vi "init.vi"(8 "error in (no error)":errorcluster, 10 "Torque Value":refnum<data-value>, 11 "Torque Transducer in":refnum<class "Torque Transducer.lvclass">) -> (0 "error out":errorcluster, 3 "Torque Transducer out":refnum<class "Torque Transducer.lvclass">)   [LabVIEW 2025, in "Torque Transducer.lvclass"]
uses:
  Torque Transducer.lvclass
  Torque Transducer.lvclass/Torque Transducer.ctl
  <vilib>/DAQmx/create/channels.llb/DAQmx Create Channel (AI-Torque-Bridge-Two-Point-Linear).vi
  <vilib>/DAQmx/configure/timing.llb/DAQmx Timing (Sample Clock).vi
panel:
  in  "units":i32(ring)=15882 items=["Nm"=15881, "oz-in"=15882, "lb-in"=15883, "lb-ft"=15884, "From Custom Scale"=10065]
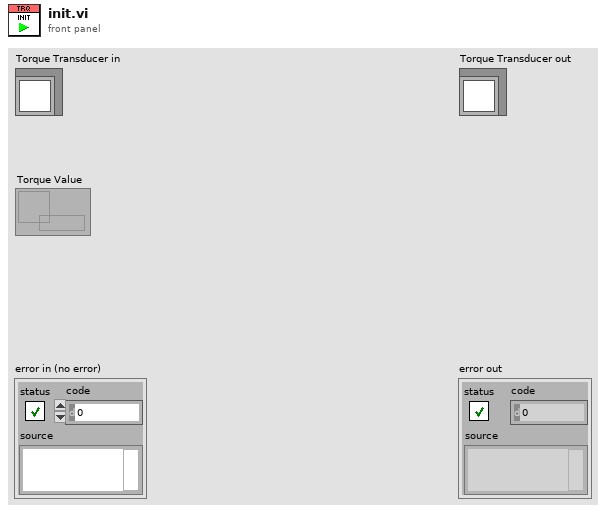
[diagram p1: front panel]
types:
  T1 = cluster{"first electrical value":dbl, "second electrical value":dbl, "electrical units":i32, "first physical value":dbl, "second physical value":dbl, "physical units":i32}
  T2 = cluster{"bridge configuration":i32, "voltage excitation source":i32, "voltage excitation value":dbl, "nominal bridge resistance":dbl}
  T3 = typedef "LVStringsAndValuesArrayTypeDef_I32.ctl" = cluster{"String":string, "Value":i32}[]
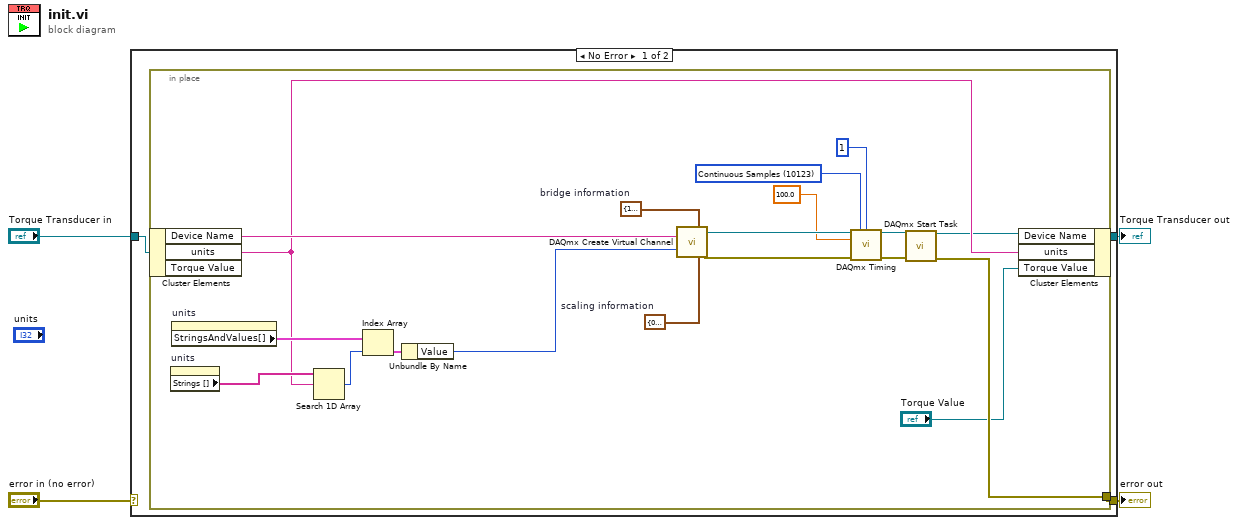
[diagram p0: block diagram]
diagram:
  n1 = case shown="No Error" "error in (no error)" {
    selector: "error in (no error)" -> [_ w28]
    tunnel: [w5 w28] -> w3
    tunnel: [w6 w27] -> w1
    tunnel: "Torque Transducer in" -> [w7 w27]
    frame No Error {
      n2 = in-place {
        in-place-border: [w9] -> w5
        w12 = 10123 items=["Finite Samples"=10178, "Continuous Samples"=10123, "Hardware Timed Single Point"=12522] ("sample mode")
        w19 = T1 {"first electrical value"=0.0, "second electrical value"=5.0, "electrical units"=15897, "first physical value"=0.0, "second physical value"=200.0, "physical units"=15883}  # scaling information
        w20 = T2 {"bridge configuration"=10182, "voltage excitation source"=10200, "voltage excitation value"=2.5, "nominal bridge resistance"=350.0}  # bridge information
        n3 = in-place-cluster #1(w7) -> ("Device Name"=w26:string, "units"=w18:string)  [unwired: 1 out]
        n4 = property on="units" class="Ring (strict)"() -> ("Strings []"=w25:string[])  [unwired: 2 in, 2 out]
        n5 = property on="units" class="Ring (strict)"() -> ("StringsAndValues[]"=w24:T3)  [unwired: 2 in, 2 out]
        n6 = Search 1D Array(1D array=w25, element=w18) -> (index of element=w23:i32)  [unwired: 1 in]
        n7 = Index Array(array=w24, index=w23) -> (element=w22:cluster{"String":string, "Value":i32})
        n8 = Unbundle By Name(w22) -> ("Value"=w21:i32)
        n9 = call-poly <vilib>:"DAQmx Create Virtual Channel.vi"("bridge information"=w20, "physical channels"=w26, "units"=w21, "scaling information"=w19) -> ("task out"=w15:refnum<k21>, "error out"=w14:errorcluster)  [unwired: 10 in]
        n10 = call-poly <vilib>:"DAQmx Timing.vi"("task/channels in"=w15, "sample mode"=w12, "samples per channel"=1, "rate"=100.0, "error in"=w14) -> ("task out"=w17:refnum<k21>, "error out"=w16:errorcluster)  [unwired: 9 in]
        n11 = call <vilib>:"DAQmx Start Task.vi"("task/channels in"=w17, "error in"=w16) -> ("task out"=w10:refnum<k21>, "error out"=w9:errorcluster)  [unwired: 12 in]
        n12 = in-place-cluster #1("Device Name"=w10, "units"=w18, "Torque Value"="Torque Value") -> (w6:refnum<class "Torque Transducer.lvclass">)
      }
    }
    frame Error {
    }
  }
  "error out" <- w3
  "Torque Transducer out" <- w1
